vi "Frames.Refs.Cleanup.vi"(11 "Lookup":variant) -> (0 "Array":errorcluster[](array[cluster]))   [LabVIEW 2024, in "Diagnostics Addon Engine.lvlib"]
uses:
  Diagnostics Addon Engine.lvlib
  Addon Shared/SubVIs/Constants.vi
  Addon Shared/Diagnostics Addon Shared.lvlib
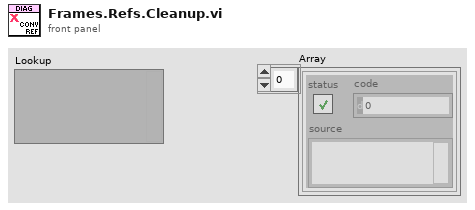
[diagram p1: front panel]
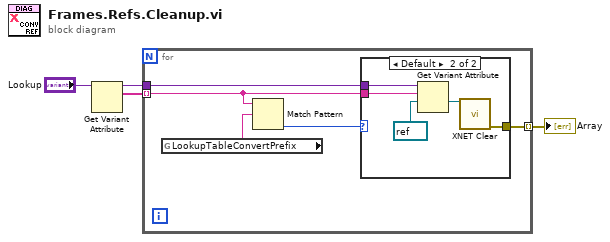
[diagram p0: block diagram]
diagram:
  n1 = Get Variant Attribute(Variant="Lookup") -> (duplicate Variant=w3:variant, names=w2:string[])  [unwired: 3 in, 2 out]
  n2 = for {
    tunnel: [w9] -> w1 mode=indexing
    tunnel: w3 -> [w8]
    tunnel: w2 -> [w5] mode=indexing
    n3 = global read "Constants.vi" "LookupTableConvertPrefix"() -> (w7:string)
    n4 = Match Pattern(string=w5, regular expression=w7) -> (offset past match=w6:i32)  [unwired: 1 in, 3 out]
    n5 = case shown="Default" w6 {
      tunnel: [_ w14] -> w9
      tunnel: w8 -> [_ w11]
      tunnel: w5 -> [_ w10]
      frame -1 {
      }
      frame Default {
        n6 = Get Variant Attribute(Variant=w11, name=w10, default value (empty Variant)=refnum<k21> refnum ("DID Conversion")) -> (value=w12:refnum<k21>)  [unwired: 1 in, 3 out]
        n7 = call <vilib>:"XNET Clear.vi"("session in"=w12) -> ("error out"=w14:errorcluster)  [unwired: 14 in]
      }
    }
  }
  "Array" <- w1
